vi "Read Block Values.vi"(8 "error in (no error)":errorcluster, 9 "Read Length":i32, 10 "Start Index":i32, 11 "Virtual Memory Unit in":refnum<class "Virtual Memory Unit.lvclass">) -> (0 "error out":errorcluster, 2 "Read Block":u16[](array[numeric]) format="%04x")   [LabVIEW 2020, in "BCI-1553 API.lvlib" / "Virtual Memory.lvlib" / "Virtual Memory Unit.lvclass"]
doc: "Reads a contiguous block of values from the memory."
uses:
  Virtual Memory Unit.lvclass
  Virtual Memory Unit.lvclass/Virtual Memory Unit.ctl
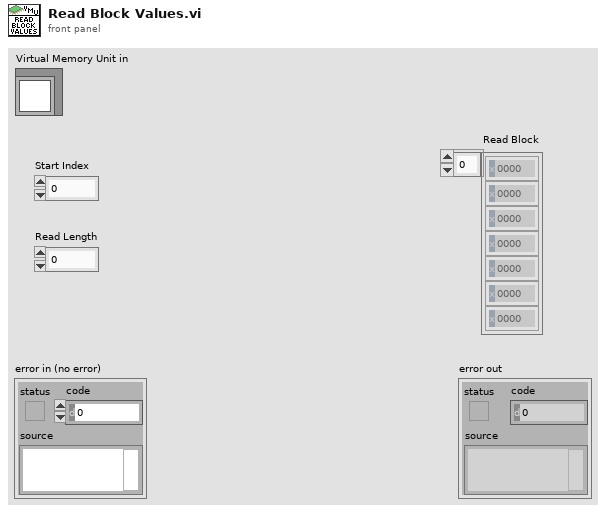
[diagram p1: front panel]
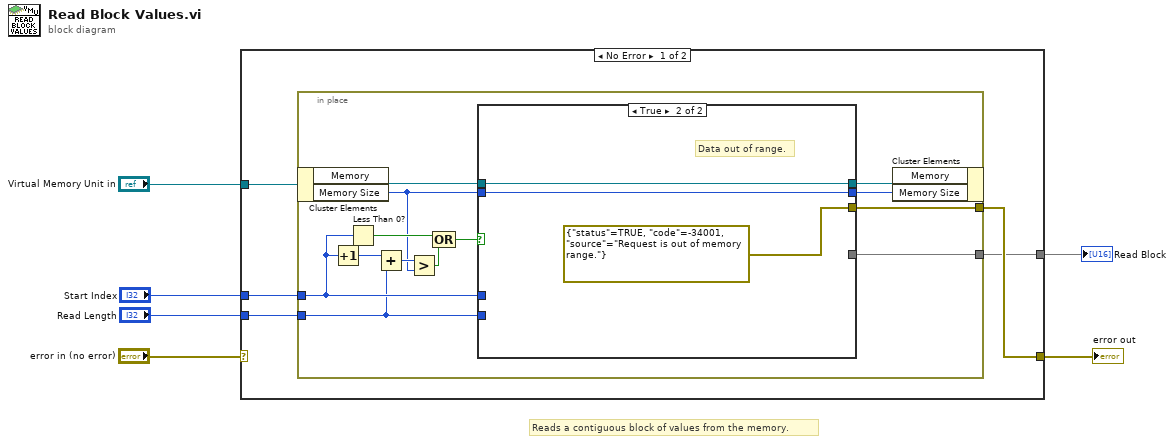
[diagram p0: block diagram]
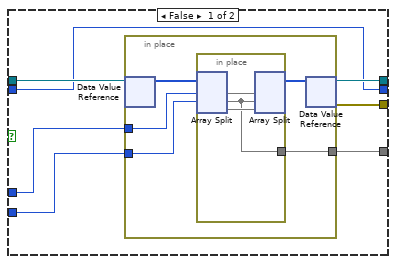
[diagram p2: hidden frame]
diagram:
  # "Reads a contiguous block of values from the memory."
  n1 = case shown="No Error" "error in (no error)" {
    selector: "error in (no error)" -> [_ w43]
    tunnel: [w8 w43] -> w5
    tunnel: "Virtual Memory Unit in" -> [w11 _]
    tunnel: "Start Index" -> [w10 _]
    tunnel: "Read Length" -> [w9 _]
    tunnel: [w7 _] -> w1
    frame No Error {
      n2 = in-place {
        in-place-border: w10 -> [w16]
        in-place-border: w9 -> [w13]
        in-place-border: [w22] -> w8
        in-place-border: [w12] -> w7
        n3 = in-place-cluster #1(w11) -> ("Memory"=w24:refnum<data-value>, "Memory Size"=w15:i32)
        n4 = Increment(x=w16) -> (x+1=w19:i32)
        n5 = Less Than 0?(x=w16) -> (x < 0?=w18:bool)
        n6 = Add(x=w19, y=w13) -> (x+y=w21:i32)
        n7 = Greater?(x=w21, y=w15) -> (0:w17:bool)
        n8 = Compound Arithmetic op=OR(w18, w17) -> (w20:bool)
        n9 = case shown="True" w20 {
          tunnel: w24 -> [w31 w42]
          tunnel: [w30 w42] -> w23
          tunnel: [w29 errorcluster {"status"=TRUE, "code"=-34001, "source"="Request is out of memory range."} ("error IO")] -> w22
          tunnel: w16 -> [w27 _]
          tunnel: w13 -> [w26 _]
          tunnel: w15 -> [w28 w41]
          tunnel: [w28 w41] -> w14
          tunnel: [w25 _] -> w12
          frame False {
            n10 = in-place {
              in-place-border: w27 -> [w34]
              in-place-border: w26 -> [w33]
              in-place-border: [w32] -> w25
              n11 = in-place-dvr #2(w31) -> (w36:u16[])  [unwired: 1 out]
              n12 = in-place {
                in-place-border: [w37] -> w32
                n13 = in-place-split #3(w36, w34, w33) -> (w39:u16[], w37:u16[], w38:u16[])
                n14 = in-place-split #3(w39, w37, w38) -> (w35:u16[])  [unwired: 2 out]
              }
              n15 = in-place-dvr #2(w35) -> (w30:refnum<data-value>, w29:errorcluster)
            }
          }
          frame True {
            # "Data out of range."
          }
        }
        n16 = in-place-cluster #1("Memory"=w23, "Memory Size"=w14) -> ()  [unwired: 1 out]
      }
    }
    frame Error {
    }
  }
  "error out" <- w5
  "Read Block" <- w1
